vi "Read Cal Tone Pin.vi"(8 "error in (no error)":errorcluster, 11 "Scalar SA Path in":refnum<class "SA Abstract Path.lvclass">) -> (0 "error out":errorcluster, 2 "Cal Tone Pin":string, 3 "Scalar SA Path out":refnum<class "SA Abstract Path.lvclass">)   [LabVIEW 2023, in "RFFixtureCharact.Public.lvlib" / "SA Abstract Path.lvclass"]
uses:
  SA Abstract Path.lvclass
  SA Abstract Path.lvclass/SA Abstract Path.ctl
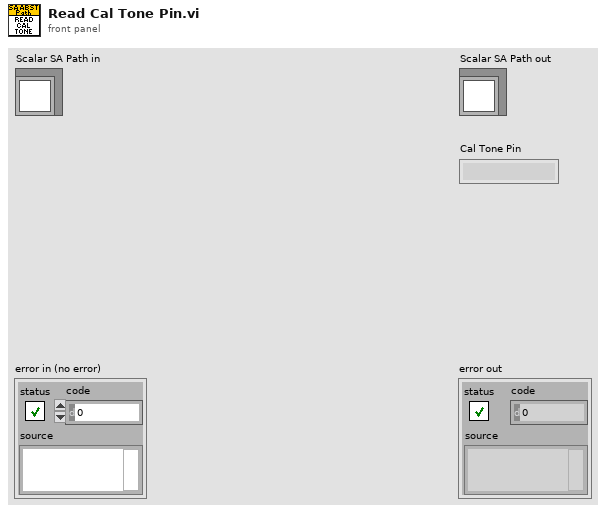
[diagram p1: front panel]
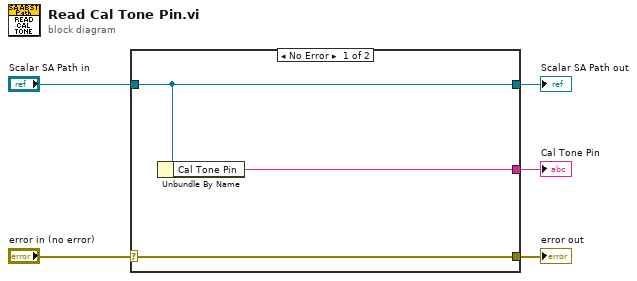
[diagram p0: block diagram]
diagram:
  n1 = case shown="No Error" "error in (no error)" {
    selector: "error in (no error)" -> [w8 w9]
    tunnel: [w8 w9] -> w4
    tunnel: [w7 w10] -> w2
    tunnel: "Scalar SA Path in" -> [w7 w10]
    tunnel: [w6 _] -> w1
    frame No Error {
      n2 = Unbundle By Name(w7) -> ("Cal Tone Pin"=w6:string)
    }
    frame Error {
    }
  }
  "error out" <- w4
  "Scalar SA Path out" <- w2
  "Cal Tone Pin" <- w1
